vi "Query Multi Eval Meas List Segment Transform Precoding.vi"(6 "BWP (0)":i32, 7 "CC (1)":T1=1, 8 "error in (no error)":errorcluster, 9 "Segment (1)":i32=1, 10 "Instance (1)":T2=1, 11 "VISA resource name":refnum<visa-resource-name>) -> (0 "error out":errorcluster, 2 "Transform Precoding":bool, 3 "VISA resource name out":refnum<visa-resource-name>)   [LabVIEW 2020, in "Rohde&Schwarz CMWXP NR FR1 Measurement.lvlib"]
doc: "Queries whether the <BWP> on carrier <cc> in segment <no> uses a transform precoding VI.\n\nAttribute:\n-\n\nRemote-control command:\nCONFigure:NRSub:MEAS<i>:LIST:SEGMent<no>[:CC<cc>]:BWPart:PUSCh:DFTPrecoding?"
uses:
  <instrlib>/Rohde&Schwarz CMWXP NR FR1 Measurement/Rohde&Schwarz CMWXP NR FR1 Measurement.lvlib
  <instrlib>/Rohde&Schwarz CMWXP NR FR1 Measurement/Private/_Instance.ctl
  <instrlib>/Rohde&Schwarz CMWXP NR FR1 Measurement/Private/_Carrier Component.ctl
  <instrlib>/Rohde&Schwarz CMWXP NR FR1 Measurement/Private/rsidr_core.llb/rsidr_core.lvlib
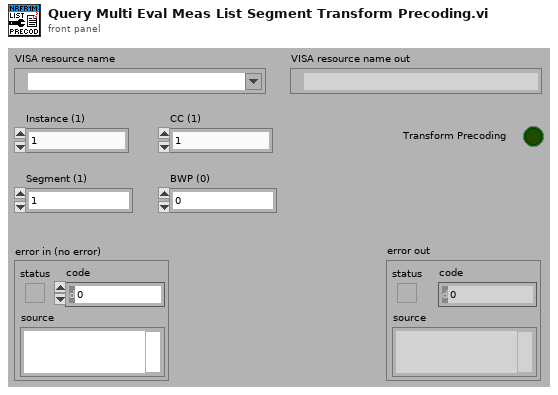
[diagram p1: front panel]
types:
  T1 = typedef "Rohde&Schwarz CMWXP NR FR1 Measurement.lvlib/_Carrier Component.ctl" = i32
  T2 = typedef "Rohde&Schwarz CMWXP NR FR1 Measurement.lvlib/_Instance.ctl" = i32
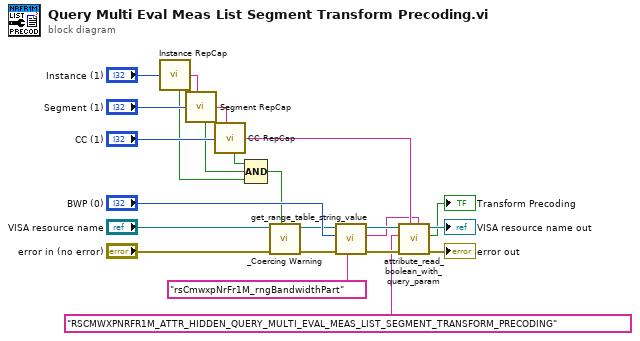
[diagram p0: block diagram]
diagram:
  n1 = call <instrlib>:"Instance RepCap.vi"("Instance In"="Instance (1)") -> ("In Range?"=w8:bool, "RepCap Identifier Out"=w20:string)  [unwired: 1 in]
  n2 = call <instrlib>:"Segment RepCap.vi"("Segment In"="Segment (1)", "RepCap String In (\"\")"=w20) -> ("In Range?"=w7:bool, "RepCap Identifier Out"=w19:string)
  n3 = call <instrlib>:"CC RepCap.vi"("CC In"="CC (1)", "RepCap String In (\"\")"=w19) -> ("In Range?"=w6:bool, "RepCap Identifier Out"=w11:string)
  n4 = Compound Arithmetic op=AND(w6, w7, w8) -> (w1:bool)
  n5 = call <instrlib>:"_Coercing Warning.vi"("In Range?"=w1, "error in (no error)"="error in (no error)", "VISA resource name"="VISA resource name") -> ("error out"=w3:errorcluster, "VISA resource name out"=w2:refnum<visa-resource-name>)  [unwired: 7 in]
  n6 = call <instrlib>:"get_range_table_string_value.vi"("Range Table ID in"="rsCmwxpNrFr1M_rngBandwidthPart", "error in"=w3, "I32 input"="BWP (0)", "VISA resource name"=w2) -> ("error out"=w16:errorcluster, "String Value out"=w10:string, "VISA resource name out"=w15:refnum<visa-resource-name>)  [unwired: 5 in]
  n7 = call <instrlib>:"attribute_read_boolean_with_query_param.vi"("Query Parameter (None)"=w10, "Repeated Capability"=w11, "error in"=w16, "Attribute ID"="RSCMWXPNRFR1M_ATTR_HIDDEN_QUERY_MULTI_EVAL_MEAS_LIST_SEGMENT_TRANSFORM_PRECODING", "VISA resource name"=w15) -> ("error out"=→"error out":errorcluster, "Boolean out"=→"Transform Precoding":bool, "VISA resource name out"=→"VISA resource name out":refnum<visa-resource-name>)  [unwired: 4 in]
